vi "NHMFL SCMPS initialize.vi"(0 "VISA session":refnum<visa-resource-name>="GPIB0::22::INSTR") -> (1 "dup VISA session":refnum<visa-resource-name>, 2 "Output Cluster":T2 {"MaxLambdaCurrent [A]" format="%.2f"; "LambdaRates [A/min]" format="%.5e"; "MaxNormalCurrent [A]" format="%.2f"; "StabilitySetting [%]" format="%.2f"; "FieldCurrentRatio [T/A]" format="%.2f"; "SwitchWaitTime [s]" format="%.2f"; "SwitchHtrCurrent [mA]" format="%.2f"; "TrainRates [A/min]" format="%.5e"; "NormalRates [A/min]" format="%.5e"; "Breakpts [A]" format="%.5e"}, 3 "Mode Out":T1(ring), 4 "Programmed Field":dbl format="%.2f", 5 "Ramp Rate":dbl format="%.2f", 6 "Persistent Field":dbl format="%.2f", 7 "Persistent":bool)   [LabVIEW 2021]
panel:
  in  "Input Cluster":T2 {"MaxLambdaCurrent [A]" format="%.2f"; "LambdaRates [A/min]" format="%.5e"; "MaxNormalCurrent [A]" format="%.2f"; "StabilitySetting [%]" format="%.2f"; "FieldCurrentRatio [T/A]" format="%.2f"; "SwitchWaitTime [s]" format="%.2f"; "SwitchHtrCurrent [mA]" format="%.2f"; "TrainRates [A/min]" format="%.5e"; "NormalRates [A/min]" format="%.5e"; "Breakpts [A]" format="%.5e"}
  out "Field":dbl format="%.2f"
  out "error out":errorcluster
  in  "error in (no error)":errorcluster
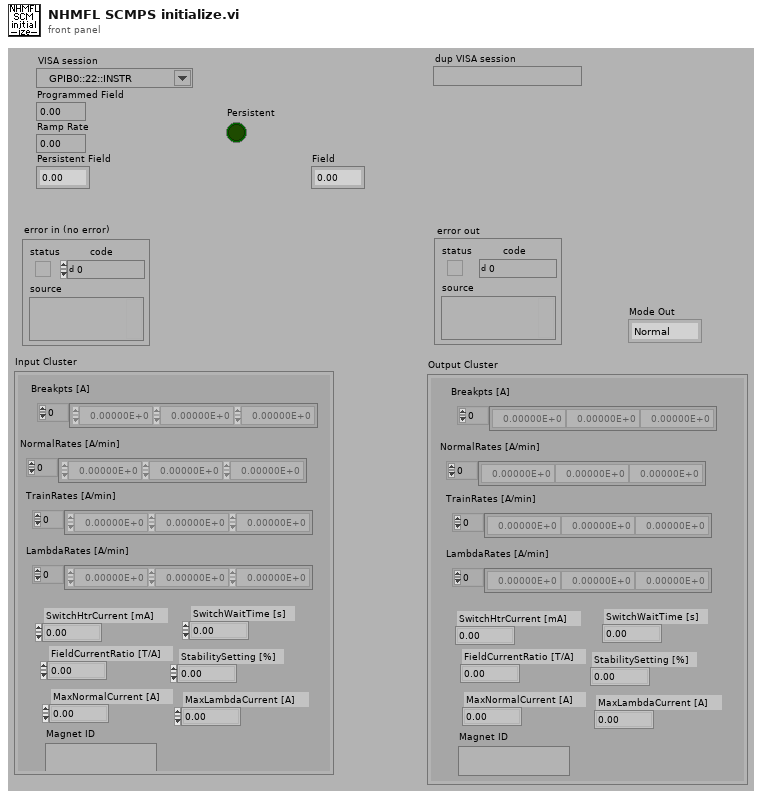
[diagram p1: front panel]
types:
  T1 = enum16{"Normal", "Train", "Lambda", "Train & Lambda"}
  T2 = cluster{"Breakpts [A]":dbl[], "NormalRates [A/min]":dbl[], "TrainRates [A/min]":dbl[], "SwitchHtrCurrent [mA]":dbl, "SwitchWaitTime [s]":dbl, "FieldCurrentRatio [T/A]":dbl, "StabilitySetting [%]":dbl, "MaxNormalCurrent [A]":dbl, "Magnet ID":string, "LambdaRates [A/min]":dbl[], "MaxLambdaCurrent [A]":dbl}
  T3 = enum16{"No Response", "Ramping to programmed field ", "Holding at programmed field", "Paused", "Ramp Manual Up", "Ramp Manual Down", "Ramping to Zero", "QUENCH", "Heating Persistence Switch", "At Zero Current"}
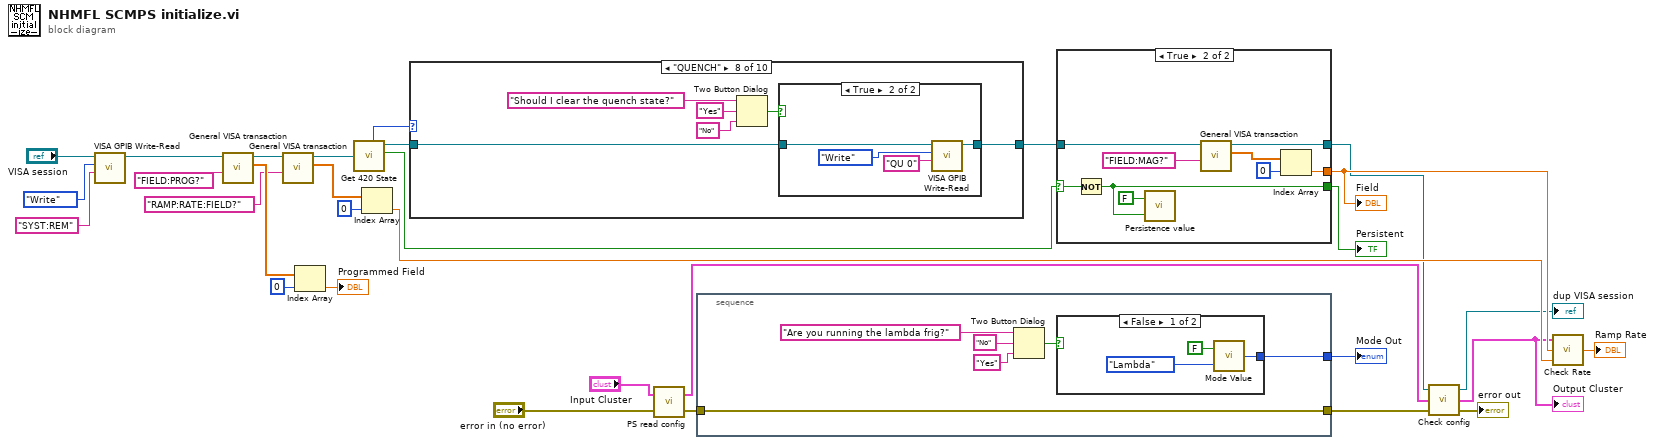
[diagram p0: block diagram]
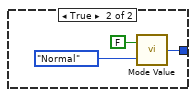
[diagram p12: hidden frame]
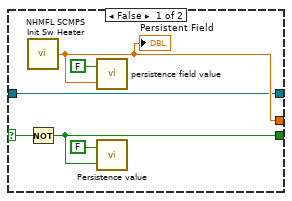
[diagram p13: hidden frame]
diagram:
  n1 = call "VISA GPIB Write-Read.vi"("Command"="SYST:REM" ("Command String"), "Action"=enum16{"Write", "Read", "Write & Read"}."Write", "VISA resource name"="VISA session") -> ("dup VISA Session"=w9:refnum<visa-resource-name>)  [unwired: 5 in, 3 out]
  n2 = call "General VISA transaction.vi"("Command String"="FIELD:PROG?", "VISA Session"=w9) -> ("Measurement"=w30:dbl[], "dup VISA Session"=w27:refnum<visa-resource-name>)  [unwired: 4 in, 4 out]
  n3 = call "General VISA transaction.vi"("Command String"="RAMP:RATE:FIELD?", "VISA Session"=w27) -> ("Measurement"=w24:dbl[], "dup VISA Session"=w4:refnum<visa-resource-name>)  [unwired: 4 in, 4 out]
  n4 = Index Array(array=w30, index=0) -> (element=→"Programmed Field":dbl)
  n5 = call "Get 420 State.vi"("VISA session"=w4) -> ("State"=w8:T3, "dup VISA session"=w5:refnum<visa-resource-name>, "Switch Heater"=w23:bool)  [unwired: 3 out]
  n6 = Index Array(array=w24, index=0) -> (element=w19:dbl)
  n7 = case shown="\"QUENCH\"" w8 {
    tunnel: w5 -> [w32 w33 w34 w35 w36 w37 w38 w40 w50 w51]
    tunnel: [w32 w33 w34 w35 w36 w37 w38 w39 w50 w51] -> w7
    frame "No Response", Default {
    }
    frame "Holding at programmed field" {
    }
    frame "Ramping to programmed field " {
    }
    frame "Paused" {
    }
    frame "Ramp Manual Up" {
    }
    frame "Ramp Manual Down" {
    }
    frame "Ramping to Zero" {
    }
    frame "QUENCH" {
      n8 = Two Button Dialog(message="Should I clear the quench state?", 1:"No" ("F button name (\"Cancel\")"), 2:"Yes" ("T button name (\"OK\")")) -> (T button?=w41:bool)
      n9 = case shown="True" w41 {
        tunnel: w40 -> [w45 w47]
        tunnel: [w45 w46] -> w39
        frame False {
        }
        frame True {
          n10 = call "VISA GPIB Write-Read.vi"("Command"="QU 0" ("Command String"), "Action"=enum16{"Write", "Read", "Write & Read"}."Write", "VISA resource name"=w47) -> ("dup VISA Session"=w46:refnum<visa-resource-name>)  [unwired: 5 in, 3 out]
        }
      }
    }
    frame "Heating Persistence Switch" {
    }
    frame "At Zero Current" {
    }
  }
  n11 = call "PS read config.vi"("error in (no error)"="error in (no error)", "Input Cluster"="Input Cluster") -> ("error out"=w16:errorcluster, "output cluster"=w1:T2)
  n12 = stacked-sequence {
    tunnel: w16 -> [w53]
    tunnel: [w53] -> w15
    tunnel: [w52] -> w12
    frame #0 {
      n13 = Two Button Dialog(message="Are you running the lambda frig?", 1:"Yes" ("F button name (\"Cancel\")"), 2:"No" ("T button name (\"OK\")")) -> (T button?=w54:bool)
      n14 = case shown="False" w54 {
        tunnel: [w58 w61] -> w52
        frame False {
          n15 = call "Mode Value.vi"("Mode In"=T1."Lambda", "Read/Write this vi"=FALSE) -> ("Mode Out"=w58:T1)
        }
        frame True {
          n16 = call "Mode Value.vi"("Mode In"=T1."Normal", "Read/Write this vi"=FALSE) -> ("Mode Out"=w61:T1)
        }
      }
    }
  }
  "Mode Out" <- w12
  n17 = case shown="True" w23 {
    selector: w23 -> [w66 w77]
    tunnel: [w65 w76] -> w22
    tunnel: w7 -> [w64 w72]
    tunnel: [w69 w71] -> w17
    tunnel: [w64 w70] -> w3
    frame False {
      n18 = call "NHMFL SCMPS Init Sw Heater.vi"() -> ("Persistent Field"=w69:dbl)  [unwired: 1 in]
      "Persistent Field" <- w69
      n19 = Not(x=w66) -> (.not. x?=w65:bool)
      n20 = call "persistence field value.vi"("Persistent Field In"=w69, "Read/Write this vi"=FALSE) -> ()  [unwired: 1 out]
      n21 = call "Persistence value.vi"("Persistence In"=w65, "Read/Write this vi"=FALSE) -> ()  [unwired: 1 out]
    }
    frame True {
      n22 = Not(x=w77) -> (.not. x?=w76:bool)
      n23 = call "Persistence value.vi"("Persistence In"=w76, "Read/Write this vi"=FALSE) -> ()  [unwired: 1 out]
      n24 = call "General VISA transaction.vi"("Command String"="FIELD:MAG?", "VISA Session"=w72) -> ("Measurement"=w74:dbl[], "dup VISA Session"=w70:refnum<visa-resource-name>)  [unwired: 4 in, 4 out]
      n25 = Index Array(array=w74, index=0) -> (element=w71:dbl)
    }
  }
  "Persistent" <- w22
  "Field" <- w17
  n26 = call "Check config.vi"("error in (no error)"=w15, "input cluster"=w1, "VISA session"=w3) -> ("error out"=→"error out":errorcluster, "output cluster"=w14:T2, "VISA session dup"=→"dup VISA session":refnum<visa-resource-name>)
  "Output Cluster" <- w14
  n27 = call "Check Rate.vi"("Rate"=w19, "Field"=w17, "input cluster"=w14) -> ("Checked Rate"=→"Ramp Rate":dbl)
